vi "Update GPIO Override Cache.vi"(0 "override gpio bank serdes id":T2, 5 "override gpio bank":T1, 7 "override gpio bank output enable":T1) -> (4 "gpio override cache":T3[](array[typedef]), 15 "valid override serdes id":bool)   [LabVIEW 2020, in "GettingStarted_Common_148X_FPGA.lvlib"]
uses:
  GettingStarted_Common_148X_FPGA.lvlib
  Types/GPIO Bank Output Configuration.ctl
  <instrlib>/FlexRIO/CSI-2/v2/FPGA/Types/GPIO Bank.ctl
  Types/SerDes Identifier.ctl
  <instrlib>/FlexRIO/CSI-2/v2/FPGA/NI CSI-2 API FPGA v2.lvlib
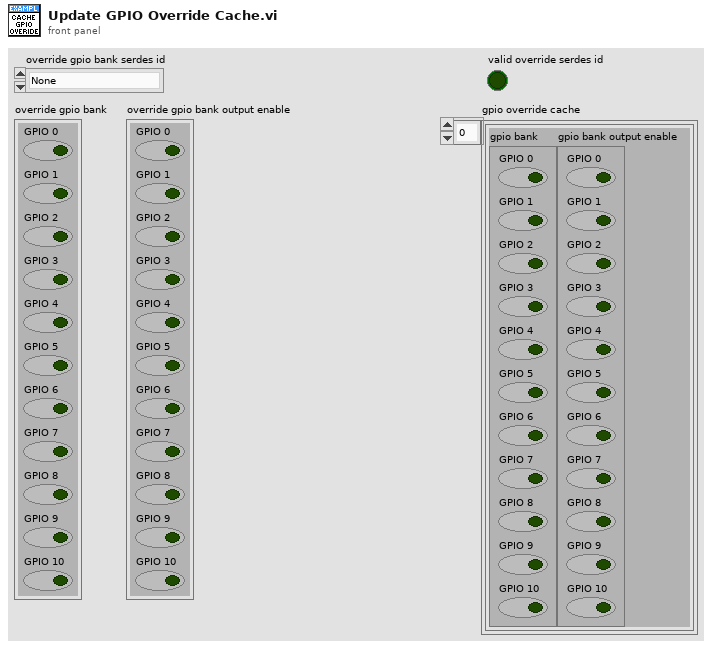
[diagram p1: front panel]
types:
  T1 = typedef "NI CSI-2 API FPGA v2.lvlib/GPIO Bank.ctl" = cluster{"GPIO 0":bool, "GPIO 1":bool, "GPIO 2":bool, "GPIO 3":bool, "GPIO 4":bool, "GPIO 5":bool, "GPIO 6":bool, "GPIO 7":bool, "GPIO 8":bool, "GPIO 9":bool, "GPIO 10":bool}
  T2 = typedef "GettingStarted_Common_148X_FPGA.lvlib/SerDes Identifier.ctl" = enum8{"None", "SI 0 Deserializer", "SI 1 Deserializer", "SI 2 Deserializer", "SI 3 Deserializer", "SI 4 Deserializer", "SI 5 Deserializer", "SI 6 Deserializer", "SI 7 Deserializer", "SO 0 Serializer", "SO 1 Serializer", "SO 2 Serializer", "SO 3 Serializer", "SO 4 Serializer", "SO 5 Serializer", "SO 6 Serializer", "SO 7 Serializer", "SI 0 SI 1 Deserializer", "SI 2 SI 3 Deserializer", "SI 4 SI 5 Deserializer", "SI 6 SI 7 Deserializer"}
  T3 = typedef "GettingStarted_Common_148X_FPGA.lvlib/GPIO Bank Output Configuration.ctl" = cluster{"gpio bank":T1, "gpio bank output enable":T1}
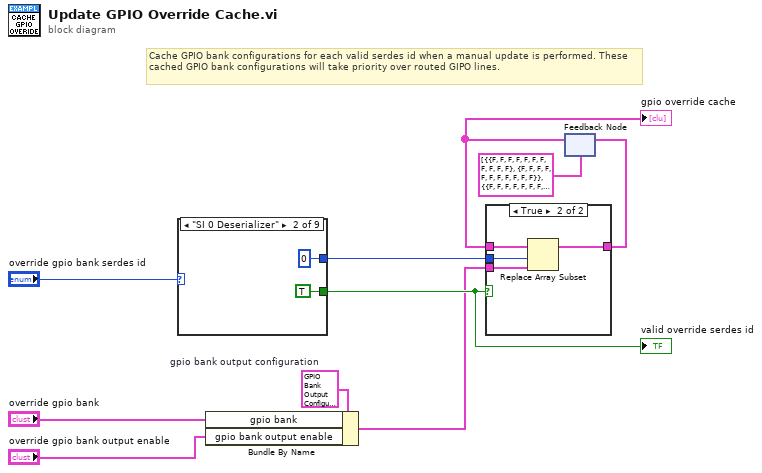
[diagram p0: block diagram]
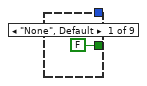
[diagram p3: hidden frame]
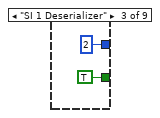
[diagram p4: hidden frame]
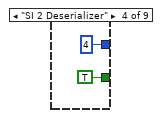
[diagram p5: hidden frame]
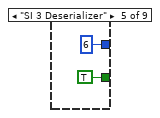
[diagram p6: hidden frame]
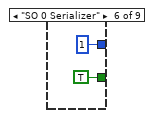
[diagram p7: hidden frame]
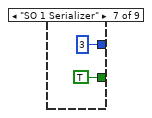
[diagram p8: hidden frame]
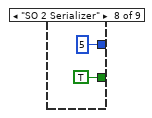
[diagram p9: hidden frame]
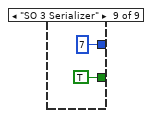
[diagram p10: hidden frame]
diagram:
  w5 = T3 {"gpio bank"={"GPIO 0"=FALSE, "GPIO 1"=FALSE, "GPIO 2"=FALSE, "GPIO 3"=FALSE, "GPIO 4"=FALSE, "GPIO 5"=FALSE, "GPIO 6"=FALSE, "GPIO 7"=FALSE, "GPIO 8"=FALSE, "GPIO 9"=FALSE, "GPIO 10"=FALSE}, "gpio bank output enable"={"GPIO 0"=FALSE, "GPIO 1"=FALSE, "GPIO 2"=FALSE, "GPIO 3"=FALSE, "GPIO 4"=FALSE, "GPIO 5"=FALSE, "GPIO 6"=FALSE, "GPIO 7"=FALSE, "GPIO 8"=FALSE, "GPIO 9"=FALSE, "GPIO 10"=FALSE}}  # gpio bank output configuration
  # "Cache GPIO bank configurations for each valid serdes id when a manual update is performed. These cached GPIO bank configurations will take priority over routed GIPO lines."
  n1 = case shown="\"SI 0 Deserializer\"" "override gpio bank serdes id" {
    tunnel: [FALSE TRUE TRUE TRUE TRUE TRUE TRUE TRUE TRUE] -> w9
    tunnel: [_ 0 ("index") 2 ("index") 4 ("index") 6 ("index") 1 ("index") 3 ("index") 5 ("index") 7 ("index")] -> w8
    frame "None", Default {
    }
    frame "SI 0 Deserializer" {
    }
    frame "SI 1 Deserializer" {
    }
    frame "SI 2 Deserializer" {
    }
    frame "SI 3 Deserializer" {
    }
    frame "SO 0 Serializer" {
    }
    frame "SO 1 Serializer" {
    }
    frame "SO 2 Serializer" {
    }
    frame "SO 3 Serializer" {
    }
  }
  "valid override serdes id" <- w9
  n2 = Bundle By Name(cluster=w5, "gpio bank"="override gpio bank", "gpio bank output enable"="override gpio bank output enable") -> (w4:T3)
  n3 = feedback #1(T3[] [{"gpio bank"={"GPIO 0"=FALSE, "GPIO 1"=FALSE, "GPIO 2"=FALSE, "GPIO 3"=FALSE, "GPIO 4"=FALSE, "GPIO 5"=FALSE, "GPIO 6"=FALSE, "GPIO 7"=FALSE, "GPIO 8"=FALSE, "GPIO 9"=FALSE, "GPIO 10"=FALSE}, "gpio bank output enable"={"GPIO 0"=FALSE, "GPIO 1"=FALSE, "GPIO 2"=FALSE, "GPIO 3"=FALSE, "GPIO 4"=FALSE, "GPIO 5"=FALSE, "GPIO 6"=FALSE, "GPIO 7"=FALSE, "GPIO 8"=FALSE, "GPIO 9"=FALSE, "GPIO 10"=FALSE}}, {"gpio bank"={"GPIO 0"=FALSE, "GPIO 1"=FALSE, "GPIO 2"=FALSE, "GPIO 3"=FALSE, "GPIO 4"=FALSE, "GPIO 5"=FALSE, "GPIO 6"=FALSE, "GPIO 7"=FALSE, "GPIO 8"=FALSE, "GPIO 9"=FALSE, "GPIO 10"=FALSE}, "gpio bank output enable"={"GPIO 0"=FALSE, "GPIO 1"=FALSE, "GPIO 2"=FALSE, "GPIO 3"=FALSE, "GPIO 4"=FALSE, "GPIO 5"=FALSE, "GPIO 6"=FALSE, "GPIO 7"=FALSE, "GPIO 8"=FALSE, "GPIO 9"=FALSE, "GPIO 10"=FALSE}}, {"gpio bank"={"GPIO 0"=FALSE, "GPIO 1"=FALSE, "GPIO 2"=FALSE, "GPIO 3"=FALSE, "GPIO 4"=FALSE, "GPIO 5"=FALSE, "GPIO 6"=FALSE, "GPIO 7"=FALSE, "GPIO 8"=FALSE, "GPIO 9"=FALSE, "GPIO 10"=FALSE}, "gpio bank output enable"={"GPIO 0"=FALSE, "GPIO 1"=FALSE, "GPIO 2"=FALSE, "GPIO 3"=FALSE, "GPIO 4"=FALSE, "GPIO 5"=FALSE, "GPIO 6"=FALSE, "GPIO 7"=FALSE, "GPIO 8"=FALSE, "GPIO 9"=FALSE, "GPIO 10"=FALSE}}, {"gpio bank"={"GPIO 0"=FALSE, "GPIO 1"=FALSE, "GPIO 2"=FALSE, "GPIO 3"=FALSE, "GPIO 4"=FALSE, "GPIO 5"=FALSE, "GPIO 6"=FALSE, "GPIO 7"=FALSE, "GPIO 8"=FALSE, "GPIO 9"=FALSE, "GPIO 10"=FALSE}, "gpio bank output enable"={"GPIO 0"=FALSE, "GPIO 1"=FALSE, "GPIO 2"=FALSE, "GPIO 3"=FALSE, "GPIO 4"=FALSE, "GPIO 5"=FALSE, "GPIO 6"=FALSE, "GPIO 7"=FALSE, "GPIO 8"=FALSE, "GPIO 9"=FALSE, "GPIO 10"=FALSE}}, {"gpio bank"={"GPIO 0"=FALSE, "GPIO 1"=FALSE, "GPIO 2"=FALSE, "GPIO 3"=FALSE, "GPIO 4"=FALSE, "GPIO 5"=FALSE, "GPIO 6"=FALSE, "GPIO 7"=FALSE, "GPIO 8"=FALSE, "GPIO 9"=FALSE, "GPIO 10"=FALSE}, "gpio bank output enable"={"GPIO 0"=FALSE, "GPIO 1"=FALSE, "GPIO 2"=FALSE, "GPIO 3"=FALSE, "GPIO 4"=FALSE, "GPIO 5"=FALSE, "GPIO 6"=FALSE, "GPIO 7"=FALSE, "GPIO 8"=FALSE, "GPIO 9"=FALSE, "GPIO 10"=FALSE}}, {"gpio bank"={"GPIO 0"=FALSE, "GPIO 1"=FALSE, "GPIO 2"=FALSE, "GPIO 3"=FALSE, "GPIO 4"=FALSE, "GPIO 5"=FALSE, "GPIO 6"=FALSE, "GPIO 7"=FALSE, "GPIO 8"=FALSE, "GPIO 9"=FALSE, "GPIO 10"=FALSE}, "gpio bank output enable"={"GPIO 0"=FALSE, "GPIO 1"=FALSE, "GPIO 2"=FALSE, "GPIO 3"=FALSE, "GPIO 4"=FALSE, "GPIO 5"=FALSE, "GPIO 6"=FALSE, "GPIO 7"=FALSE, "GPIO 8"=FALSE, "GPIO 9"=FALSE, "GPIO 10"=FALSE}}, {"gpio bank"={"GPIO 0"=FALSE, "GPIO 1"=FALSE, "GPIO 2"=FALSE, "GPIO 3"=FALSE, "GPIO 4"=FALSE, "GPIO 5"=FALSE, "GPIO 6"=FALSE, "GPIO 7"=FALSE, "GPIO 8"=FALSE, "GPIO 9"=FALSE, "GPIO 10"=FALSE}, "gpio bank output enable"={"GPIO 0"=FALSE, "GPIO 1"=FALSE, "GPIO 2"=FALSE, "GPIO 3"=FALSE, "GPIO 4"=FALSE, "GPIO 5"=FALSE, "GPIO 6"=FALSE, "GPIO 7"=FALSE, "GPIO 8"=FALSE, "GPIO 9"=FALSE, "GPIO 10"=FALSE}}, {"gpio bank"={"GPIO 0"=FALSE, "GPIO 1"=FALSE, "GPIO 2"=FALSE, "GPIO 3"=FALSE, "GPIO 4"=FALSE, "GPIO 5"=FALSE, "GPIO 6"=FALSE, "GPIO 7"=FALSE, "GPIO 8"=FALSE, "GPIO 9"=FALSE, "GPIO 10"=FALSE}, "gpio bank output enable"={"GPIO 0"=FALSE, "GPIO 1"=FALSE, "GPIO 2"=FALSE, "GPIO 3"=FALSE, "GPIO 4"=FALSE, "GPIO 5"=FALSE, "GPIO 6"=FALSE, "GPIO 7"=FALSE, "GPIO 8"=FALSE, "GPIO 9"=FALSE, "GPIO 10"=FALSE}}]) -> (w1:T3[])
  "gpio override cache" <- w1
  n4 = case shown="True" w9 {
    tunnel: [w28 w32] -> w3
    tunnel: w1 -> [w28 w31]
    tunnel: w8 -> [_ w30]
    tunnel: w4 -> [_ w29]
    frame False {
    }
    frame True {
      n5 = Replace Array Subset(array=w31, new element=w29, index=w30) -> (w32:T3[])
    }
  }
  n6 = feedback-in #1(w3) -> ()
